vi "Serial Read IMU.vi"(8 "Timeout (ms) (-1: no timeout)":i32=-1, 9 "Bytes to Read":u32, 10 "error in (no error)":errorcluster, 11 "FPGA VI Reference In":refnum<k20>) -> (0 "String":string, 2 "error out":errorcluster, 3 "FPGA VI Reference Out":refnum<k20>)   [LabVIEW 2016]
uses:
  <vilib>/rvi/errors/niLvFpgaAdjustHostInterfaceError.vi
  <vilib>/rvi/interface/nirviReadWriteControl/nirviReadWriteControl.xnode
  <vilib>/rvi/interface/Simulation/niFpgaSimulationCallBeginRW.vi
  NiFpgaLv.dll
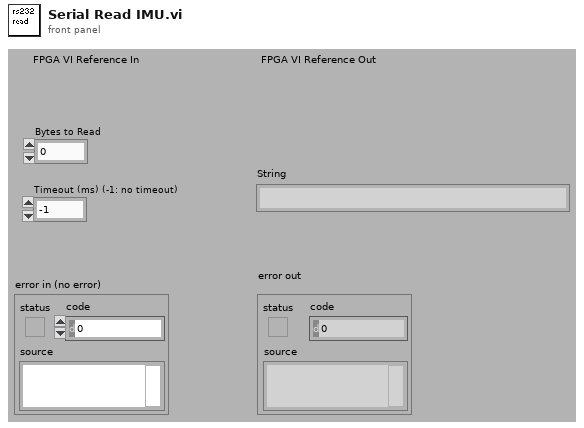
[diagram p1: front panel]
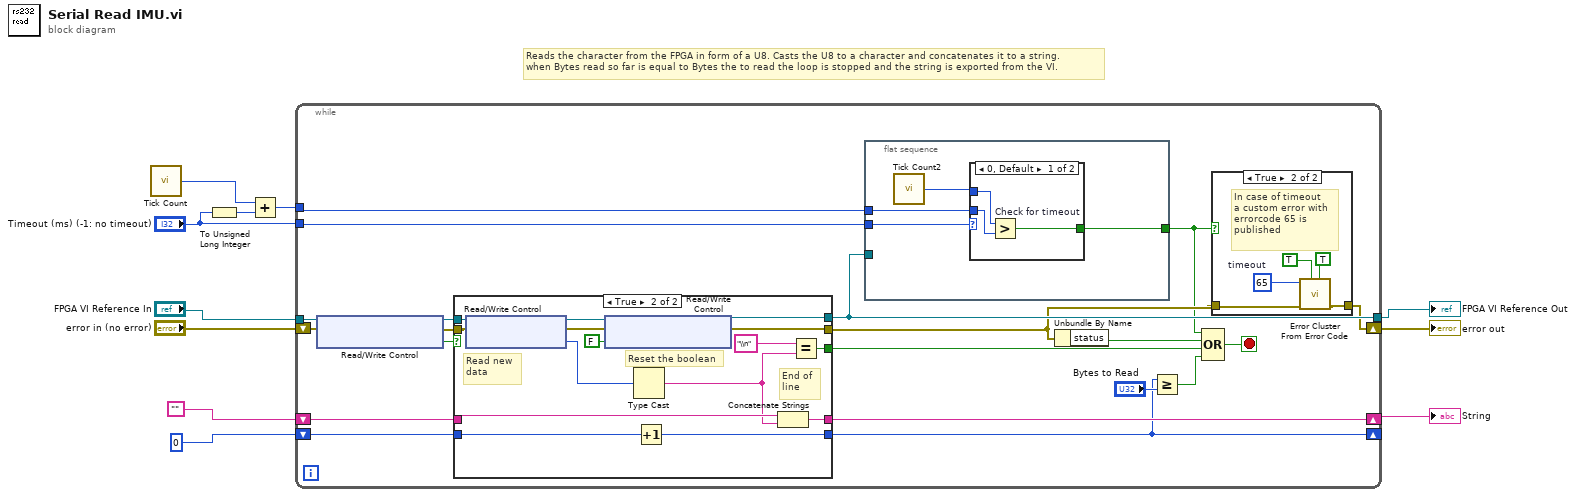
[diagram p0: block diagram]
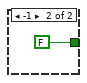
[diagram p3: hidden frame]
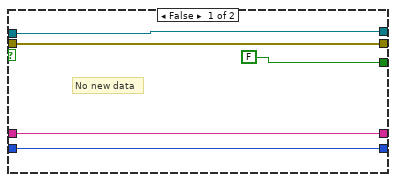
[diagram p4: hidden frame]
diagram:
  # "Reads the character from the FPGA in form of a U8. Casts the U8 to a character and concatenates it to a string.\nwhen Bytes read so far is equal to Bytes the to read the loop is stopped and the string is exported from the VI."
  n1 = call "Tick Count"() -> ("Tick Count(mSec)"=w5:u32)
  n2 = To Unsigned Long Integer(number="Timeout (ms) (-1: no timeout)") -> (unsigned 32bit integer=w4:u32)
  n3 = Add(x=w5, y=w4) -> (x+y=w6:u32)
  n4 = while {
    tunnel: "FPGA VI Reference In" -> [w15]
    tunnel: [w27] -> w1
    shift-right: [w26] -> _
    shift-left: u32 0 -> [w31]
    shift-right: [w29] -> w7
    shift-left: "" -> [w30]
    shift-right: [w19] -> w10
    shift-left: "error in (no error)" -> [w14]
    tunnel: "Timeout (ms) (-1: no timeout)" -> [w23]
    tunnel: w6 -> [w22]
    stop <- w25 stop-if-true
    n5 = xnode "Read/Write Control"("FPGA VI Reference In"=w15, "error in"=w14) -> ("FPGA VI Reference Out"=w17:refnum<k20>, "error out"=w16:errorcluster, "Read: New IMU Data"=w13:bool)
    n6 = case shown="True" w13 {
      tunnel: [w50 w65] -> w26
      tunnel: w31 -> [w50 w64]
      tunnel: w30 -> [w49 w63]
      tunnel: [w49 w62] -> w29
      tunnel: w17 -> [w48 w60]
      tunnel: [w48 w58] -> w27
      tunnel: [FALSE w56] -> w24
      tunnel: w16 -> [w46 w54]
      tunnel: [w46 w52] -> w21
      frame False {
        # "No new data"
      }
      frame True {
        # "End of \nline"
        # "Reset the boolean"
        # "Read new \ndata"
        n7 = xnode "Read/Write Control"("FPGA VI Reference In"=w60, "error in"=w54) -> ("FPGA VI Reference Out"=w59:refnum<k20>, "error out"=w53:errorcluster, "Read: IMU Char"=w61:u8)
        n8 = xnode "Read/Write Control"("FPGA VI Reference In"=w59, "error in"=w53, "Read: New IMU Data"=FALSE ("Data Read")) -> ("FPGA VI Reference Out"=w58:refnum<k20>, "error out"=w52:errorcluster)
        n9 = Type Cast(x=w61) -> (*(type *) &x=w55:string)  [unwired: 1 out]
        n10 = Increment(x=w64) -> (x+1=w65:u32)
        n11 = Concatenate Strings(w63, w55) -> (w62:string)
        n12 = Equal?(x="\\n", y=w55) -> (x = y?=w56:bool)
      }
    }
    n13 = flat-sequence {
      tunnel: w27 -> [_]
      tunnel: [w41] -> w12
      tunnel: w23 -> [w40]
      tunnel: w22 -> [w39]
      frame #0 {
        n14 = call "Tick Count2"() -> ("Tick Count(mSec)"=w38:u32)
        n15 = case shown="0, Default" w40 {
          tunnel: [w42 FALSE] -> w41
          tunnel: w39 -> [w43 _]
          tunnel: w38 -> [w44 _]
          frame 0, Default {
            n16 = Greater? "Check for timeout"(x=w44, y=w43) -> (0:w42:bool)
          }
          frame -1 {
          }
        }
      }
    }
    n17 = Unbundle By Name(w21) -> ("status"=w20:bool)
    n18 = Greater Or Equal?(x=w26, y="Bytes to Read") -> (x >= y?=w18:bool)
    n19 = Compound Arithmetic op=OR(w12, w20, w24, w18) -> (w25:bool)
    n20 = case shown="True" w12 {
      tunnel: w21 -> [w32 w36]
      tunnel: [w32 w35] -> w19
      frame False {
      }
      frame True {
        w37 = 65  # timeout
        # "In case of timeout\na custom error with\nerrorcode 65 is \npublished"
        n21 = call <vilib>:"Error Cluster From Error Code.vi"("is warning? (False)"=TRUE, "show call chain? (False)"=TRUE, "error in (no error)"=w36, "error code (0)"=w37) -> ("error out"=w35:errorcluster)  [unwired: 5 out]
      }
    }
  }
  "error out" <- w10
  "String" <- w7
  "FPGA VI Reference Out" <- w1
